vi "重启定时单元（专用）.vi"(6 "周期":i64, 7 "定时结构名称":string, 8 "error in (no error)":errorcluster caption="错误输入（无错误）", 11 "引用-定时单元VI（专用）":refnum<vi>) -> (0 "错误输出":errorcluster, 2 "引用-定时信号？":refnum<vi>, 3 "VI引用o":refnum<vi>)   [LabVIEW 2017]
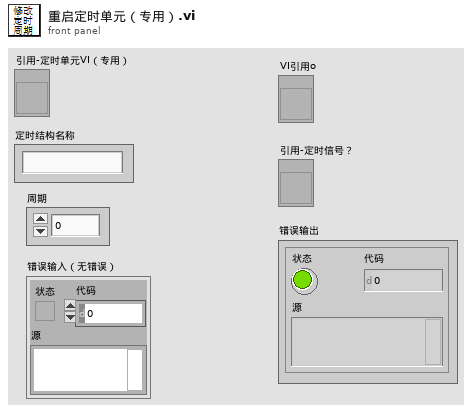
[diagram p1: front panel]
types:
  T1 = enum32{"Invalid", "Standard", "Closed", "Hidden", "Minimized", "Maximized"}
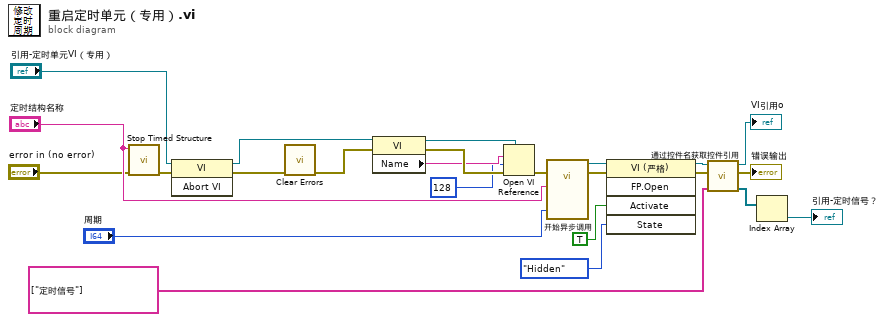
[diagram p0: block diagram]
diagram:
  n1 = call <vilib>:"Stop Timed Structure.vi"("error in (no error)"="error in (no error)", "name"="定时结构名称") -> ("error out"=w18:errorcluster)  [unwired: 9 in]
  n2 = invoke class="VI" method="Abort VI"(reference="引用-定时单元VI（专用）", error in=w18) -> (reference out=w14:refnum<vi>, error out=w17:errorcluster)  [unwired: 1 in, 1 out]
  n3 = call <vilib>:"Clear Errors.vi"("error in (no error)"=w17) -> ("error out"=w2:errorcluster)  [unwired: 5 in, 1 out]
  n4 = property class="VI"(reference=w14, error in=w2) -> (reference out=w1:refnum<vi>, error out=w15:errorcluster, "Name"=w11:string)
  n5 = Open VI Reference(type specifier VI Refnum (for type only)=w1, vi path=w11, options=128 ("选项"), error in (no error)=w15) -> (error out=w16:errorcluster)  [unwired: 2 in, 1 out]
  n6 = call-by-ref "开始异步调用"(error in=w16, "周期"="周期", "结构名称"="定时结构名称") -> (reference out=w19:refnum<vi>, error out=w21:errorcluster)  [unwired: 11 in]
  n7 = invoke class="VI (严格)" method="FP.Open"(reference=w19, error in=w21, "Activate"=TRUE ("激活？"), "State"=T1."Hidden" ("状态")) -> (reference out=w20:refnum<vi>, error out=w22:errorcluster)  [unwired: 1 in, 3 out]
  n8 = call "通过控件名获取控件引用.vi"("控件名数组"=string[] ["定时信号"], "错误输入（无错误）"=w22, "VI引用"=w20) -> ("控件引用输出"=w13:refnum<vi>[], "错误输出"=→"错误输出":errorcluster, "VI引用o"=→"VI引用o":refnum<vi>)  [unwired: 6 in]
  n9 = Index Array(array=w13) -> (element=→"引用-定时信号？":refnum<vi>)  [unwired: 1 in]
